vi "Init.vi"(8 "error in (no error)":errorcluster, 10 "_addr":u8, 11 "Motorshield in":refnum<class "Motorshield.lvclass">) -> (0 "error out":errorcluster, 3 "Motorshield out":refnum<class "Motorshield.lvclass">)   [LabVIEW 2022 SP3, in "Motorshield.lvlib" / "Motorshield.lvclass"]
uses:
  Motorshield.lvclass
  Motorshield.lvclass/Motorshield.ctl
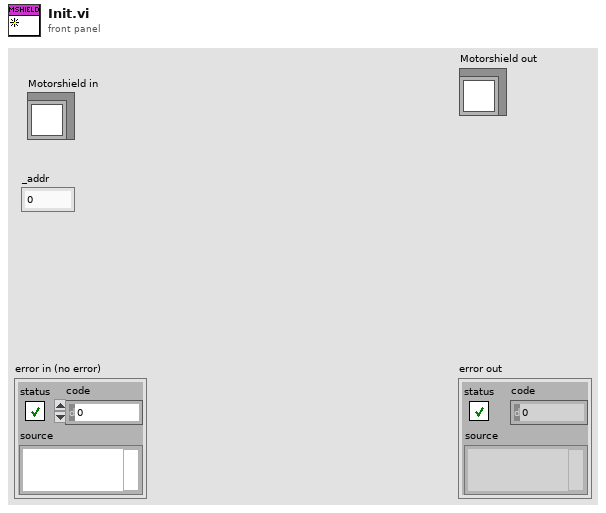
[diagram p1: front panel]
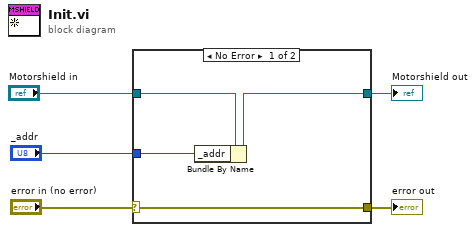
[diagram p0: block diagram]
diagram:
  n1 = case shown="No Error" "error in (no error)" {
    selector: "error in (no error)" -> [w9 w11]
    tunnel: [w9 w11] -> w4
    tunnel: [w8 w10] -> w3
    tunnel: "_addr" -> [w7 _]
    tunnel: "Motorshield in" -> [w6 w10]
    frame No Error {
      n2 = Bundle By Name(cluster=w6, "_addr"=w7) -> (w8:refnum<class "Motorshield.lvclass">)
    }
    frame Error {
    }
  }
  "error out" <- w4
  "Motorshield out" <- w3
